vi "HEWH Set Valves.vi"(0 "VISA session":refnum<visa-resource-name>="MW100", 1 "Station ID":T2=enum."A", 5 "Pressurize Tank?":bool, 7 "Valve Bank Setting":T3, 9 "Stop Intellifaucet?":bool=TRUE, 11 "Error In":errorcluster, 12 "Start Intellifaucet?":bool, 13 "Debug":bool, 14 "Refnum in":T1) -> (4 "dup VISA session":refnum<visa-resource-name>, 15 "Error Out":errorcluster)   [LabVIEW 2016]
uses:
  Type Definitions/HEWH Valve Bank Positions.ctl
  Type Definitions/Station ID Selector.ctl
  Intellifaucet/Type Definitions/INTELLIFAUCET Set Mode.ctl
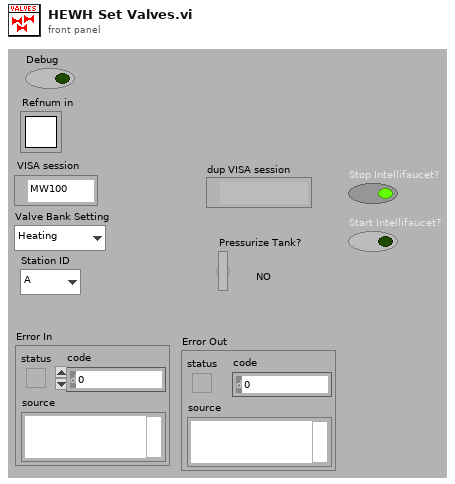
[diagram p1: front panel]
types:
  T1 = typedef "Semaphore RefNum" = refnum<k1>
  T2 = typedef "Station ID Selector.ctl" = enum16{"", "A", "B", "C", "D", "Global"}
  T3 = typedef "HEWH Valve Bank Positions.ctl" = enum16{"Heating", "Purge", "Resting", "Draw"}
  T4 = typedef "INTELLIFAUCET Set Mode.ctl" = enum16{"Adjust Temp", "Adjust Flow", "Start Flow", "Stop Flow", "Hold"}
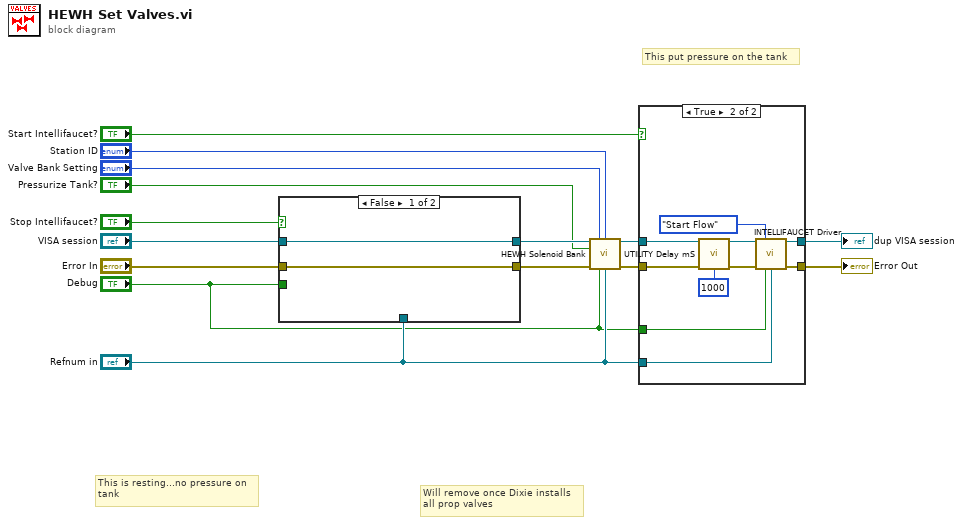
[diagram p0: block diagram]
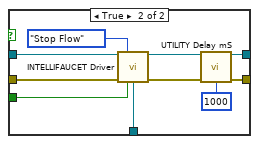
[diagram p2: hidden frame]
diagram:
  # "Will remove once Dixie installs\nall prop valves"
  # "This is resting...no pressure on\ntank"
  # "This put pressure on the tank"
  n1 = case shown="False" "Stop Intellifaucet?" {
    tunnel: [w17 w25] -> w15
    tunnel: [w16 w23] -> w5
    tunnel: "VISA session" -> [w17 w21]
    tunnel: "Error In" -> [w16 w20]
    tunnel: "Debug" -> [_ w19]
    tunnel: "Refnum in" -> [_ w18]
    frame False {
    }
    frame True {
      n2 = call "INTELLIFAUCET Driver.vi"("VISA session"=w21, "Mode"=INTELLIFAUCET_Set_Mode."Stop Flow", "Error In"=w20, "Debug"=w19, "Refnum in"=w18) -> ("VISA session out"=w25:refnum<visa-resource-name>, "Error Out"=w24:errorcluster)  [unwired: 7 in, 2 out]
      n3 = call "UTILITY Delay mS.vi"("Error In"=w24, "milliseconds to wait"=u32 1000) -> ("Error Out"=w23:errorcluster)  [unwired: 13 in]
    }
  }
  n4 = call "HEWH Solenoid Bank.vi"("VISA session"=w15, "Valve Bank Setting"="Valve Bank Setting", "Station ID"="Station ID", "Pressurize Tank?"="Pressurize Tank?", "Error In"=w5, "Debug"="Debug", "Refnum in"="Refnum in") -> ("dup VISA session"=w13:refnum<visa-resource-name>, "Error Out"=w14:errorcluster)  [unwired: 7 in]
  n5 = case shown="True" "Start Intellifaucet?" {
    tunnel: [w28 w31] -> w1
    tunnel: w14 -> [w28 w33]
    tunnel: w13 -> [w27 w36]
    tunnel: [w27 w35] -> w2
    tunnel: "Refnum in" -> [_ w30]
    tunnel: "Debug" -> [_ w29]
    frame False {
    }
    frame True {
      n6 = call "UTILITY Delay mS.vi"("Error In"=w33, "milliseconds to wait"=u32 1000) -> ("Error Out"=w32:errorcluster)  [unwired: 13 in]
      n7 = call "INTELLIFAUCET Driver.vi"("VISA session"=w36, "Mode"=INTELLIFAUCET_Set_Mode."Start Flow", "Error In"=w32, "Debug"=w29, "Refnum in"=w30) -> ("VISA session out"=w35:refnum<visa-resource-name>, "Error Out"=w31:errorcluster)  [unwired: 7 in, 2 out]
    }
  }
  "dup VISA session" <- w2
  "Error Out" <- w1
